vi "Init Image.vi"(10 "Pane Color":u32, 11 "Header Path":path) -> ()   [LabVIEW 2012]
uses:
  Image States.ctl
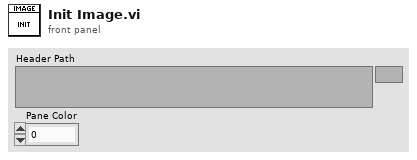
[diagram p1: front panel]
types:
  T1 = typedef "Image States.ctl" = enum16{"Init", "Print"}
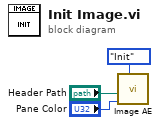
[diagram p0: block diagram]
diagram:
  n1 = call "Image AE.vi"("Image State"=Image_States."Init", "Pane Color"="Pane Color", "Header Path"="Header Path") -> ()  [unwired: 8 in, 1 out]
